vi "File_Read-Save Text.vi"(5 "Target Folder":path, 6 "Read(f) Save(t)":bool, 7 "File Name":string, 8 "Error":errorcluster, 11 "Text Data":string) -> (0 "Error Out":errorcluster, 2 "Success Out":bool, 3 "Text Data Out":string)   [LabVIEW 2020]
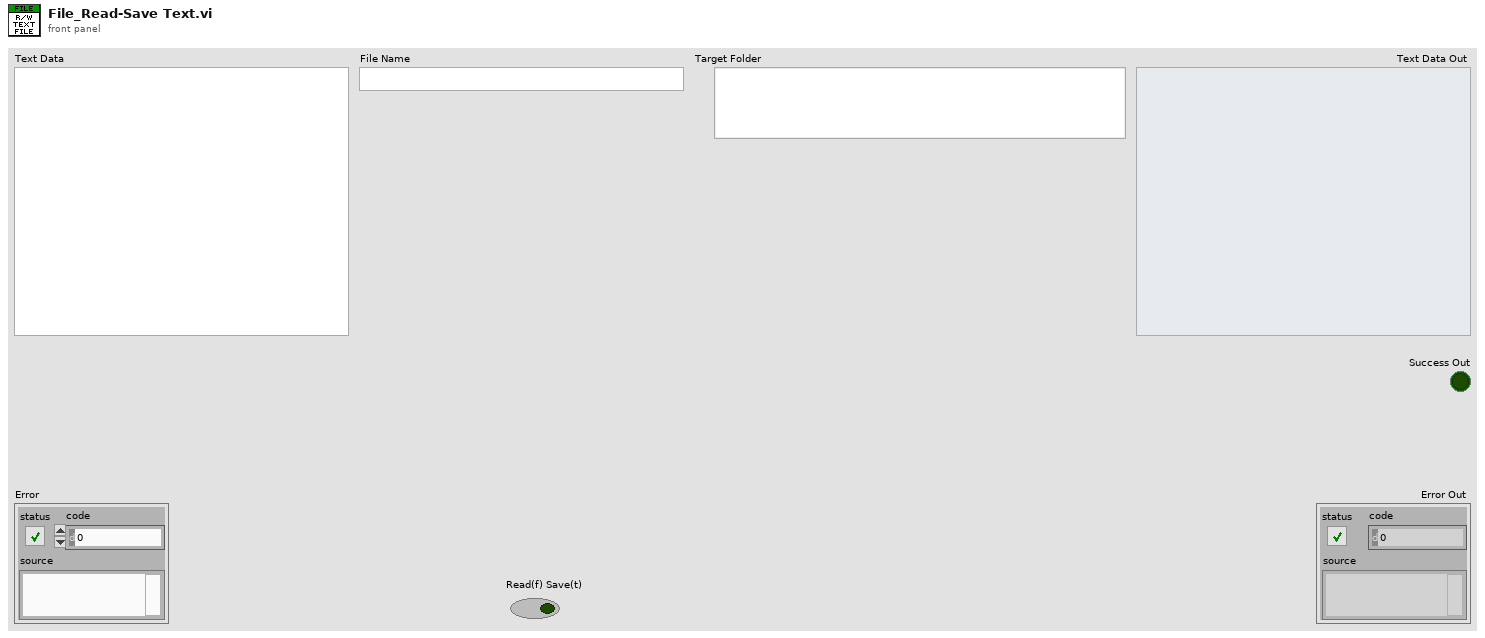
[diagram p1: front panel]
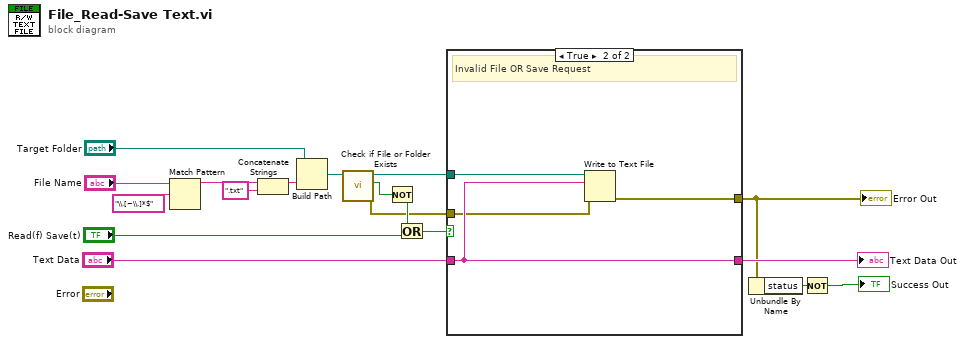
[diagram p0: block diagram]
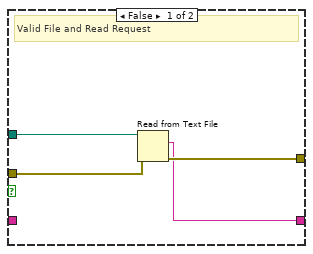
[diagram p2: hidden frame]
diagram:
  n1 = Match Pattern(string="File Name", regular expression="\\.[~\\.]*$") -> (before substring=w13:string)  [unwired: 4 out]
  n2 = Concatenate Strings(w13, ".txt" ("string")) -> (w12:string)
  n3 = Build Path(base path="Target Folder", name or relative path=w12) -> (appended path=w6:path)
  n4 = call <vilib>:"Check if File or Folder Exists.vi"("path"=w6) -> ("error out"=w1:errorcluster, "file or folder exists?"=w3:bool, "dup path"=w5:path)  [unwired: 8 in]
  n5 = Not(x=w3) -> (.not. x?=w2:bool)
  n6 = Or(x=w2, y="Read(f) Save(t)") -> (x .or. y?=w4:bool)
  n7 = case shown="True" w4 {
    tunnel: w5 -> [w20 w26]
    tunnel: "Text Data" -> [_ w24]
    tunnel: [w22 w25] -> w8
    tunnel: [w21 w24] -> w9
    tunnel: w1 -> [w19 w23]
    frame False {
      # "Valid File and Read Request"
      n8 = Read from Text File(file (use dialog)=w20, error in=w19) -> (text=w21:string, error out=w22:errorcluster)  [unwired: 2 in, 2 out]
    }
    frame True {
      # "Invalid File OR Save Request"
      n9 = Write to Text File(file (use dialog)=w26, text=w24, error in=w23) -> (error out=w25:errorcluster)  [unwired: 1 in, 2 out]
    }
  }
  "Text Data Out" <- w9
  "Error Out" <- w8
  n10 = Unbundle By Name(w8) -> ("status"=w7:bool)
  n11 = Not(x=w7) -> (.not. x?=→"Success Out":bool)
